vi "Extract 16-bit rectangle from image.vi"(2 "error in":errorcluster, 3 "AOI (t, l, b, r)":u16[](array[numeric]), 4 "Image pixel depth":u32(ring) items=["8 bits", "16 bits", "Float", "Complex", "RGB", "HSL"], 5 "Image in":T1) -> (0 "error out":errorcluster, 1 "Image Pixels (I16)":i16[][](array[numeric]))   [LabVIEW 2015]
uses:
  <vilib>/vision/Image Controls.llb/IMAQ Image.ctl
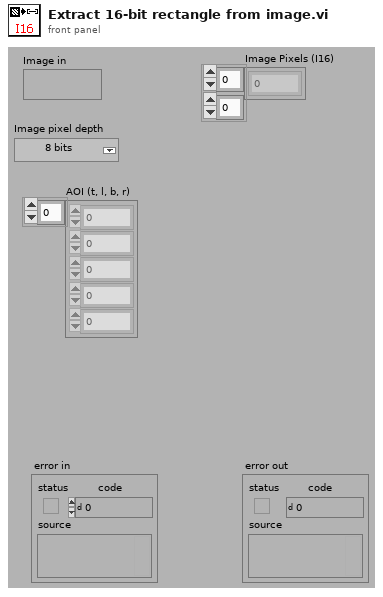
[diagram p1: front panel]
types:
  T1 = typedef "IMAQ Image.ctl" = refnum<image>
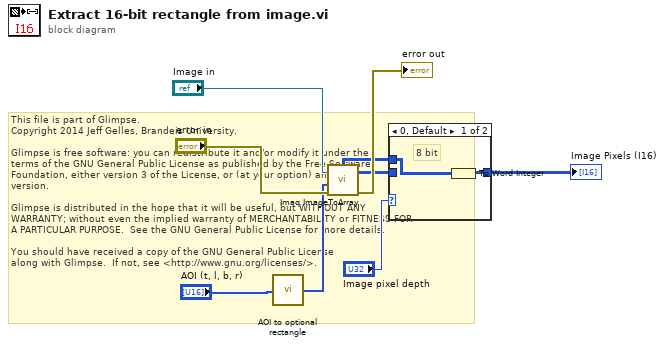
[diagram p0: block diagram]
diagram:
  # "This file is part of Glimpse. \nCopyright 2014 Jeff Gelles, Brandeis University.    \n\nGlimpse is free software: you can redistribute it and/or modify it under the \nterms of the GNU General Public License as published by the Free Software \nFoundation, either version 3 of the License, or (at your option) any later \nversion.\n\nGlimpse is distributed in the hope that it will be useful, but WITHOUT ANY \nWARRANTY; without even the implied warranty of MERCHANTABILITY or FITNESS FOR \nA PARTICULAR PURPOSE.  See the GNU General Public License for more details.\n\nYou should have received a copy of the GNU General Public License\nalong with Glimpse.  If not, see <http://www.gnu.org/licenses/>."
  n1 = call "AOI to optional rectangle.vi"("x1, y1, x2, y2 with origin (0, 0)"="AOI (t, l, b, r)") -> ("x1, y1, x2+1, y2+1 with origin (0, 0)"=w1:u16[])  [unwired: 4 out]
  n2 = call "Imaq ImageToArray"("error in (no error)"="error in", "Optional Rectangle"=w1, "Image"="Image in") -> ("error out"=→"error out":errorcluster, "Image Pixels (U8)"=w7:u8[][], "Image Pixels (I16)"=w6:i16[][])  [unwired: 3 out]
  n3 = case shown="0, Default" "Image pixel depth" {
    tunnel: [w10 w12] -> w9
    tunnel: w6 -> [_ w12]
    tunnel: w7 -> [w11 _]
    frame 0, Default {
      # "8 bit"
      n4 = To Word Integer(number=w11) -> (16bit integer=w10:i16[][])
    }
    frame 1 {
      # "16 bit"
    }
  }
  "Image Pixels (I16)" <- w9
